vi "Tran_Get (v,w).vi"(8 "error in (no error)":errorcluster, 11 "robot body ref":refnum<k20>) -> (0 "error out":errorcluster, 2 "Angular Veloctiy":sgl, 3 "Linear Velocity":sgl)   [LabVIEW 2017]
uses:
  <resource>/objmgr/LVODE.rc
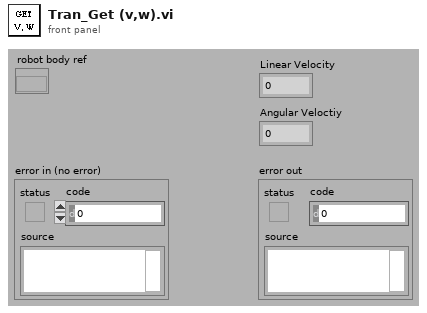
[diagram p1: front panel]
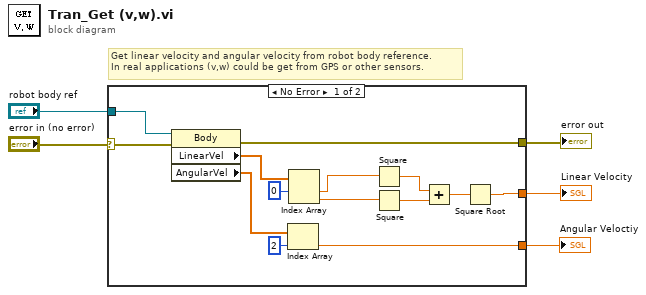
[diagram p0: block diagram]
diagram:
  # "Get linear velocity and angular velocity from robot body reference.\nIn real applications (v,w) could be get from GPS or other sensors."
  n1 = case shown="No Error" "error in (no error)" {
    selector: "error in (no error)" -> [w6 w20]
    tunnel: [w17 _] -> w5
    tunnel: [w16 _] -> w4
    tunnel: "robot body ref" -> [w8 _]
    tunnel: [w7 w20] -> w2
    frame No Error {
      n2 = property class="Body"(reference=w8, error in=w6) -> (error out=w7:errorcluster, "LinearVel"=w18:sgl[], "AngularVel"=w19:sgl[])  [unwired: 1 out]
      n3 = Index Array(array=w19, index=2) -> (element=w16:sgl)
      n4 = Index Array(array=w18, index #1=0 ("index")) -> (element #1=w11:sgl, element #2=w12:sgl)  [unwired: 1 in]
      n5 = Square(x=w11) -> (x^2=w13:sgl)
      n6 = Square(x=w12) -> (x^2=w14:sgl)
      n7 = Add(x=w13, y=w14) -> (x+y=w15:sgl)
      n8 = Square Root(x=w15) -> (sqrt(x)=w17:sgl)
    }
    frame Error {
    }
  }
  "Linear Velocity" <- w5
  "Angular Veloctiy" <- w4
  "error out" <- w2
